vi "n set piso control.vi"(8 "error in (no error)":errorcluster, 9 "l2":u16, 10 "l1":u16, 11 "n":u16) -> (0 "error out":errorcluster)   [LabVIEW 2015, in "SCANalone4x64.lvlib"]
doc: "__declspec(dllimport) void __stdcall n_set_piso_control(unsigned short n, unsigned short l1, unsigned short l2);"
uses:
  <userlib>/SCANalone4x64/SCANalone4x64.lvlib
  <userlib>/SCANalone4x64/SCANalone4x64.dll
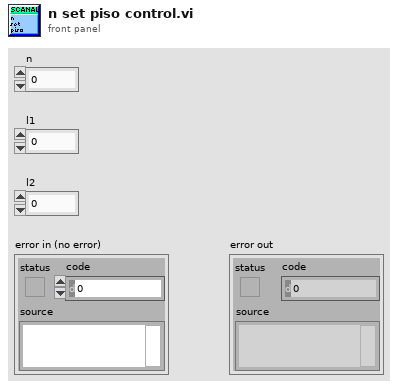
[diagram p1: front panel]
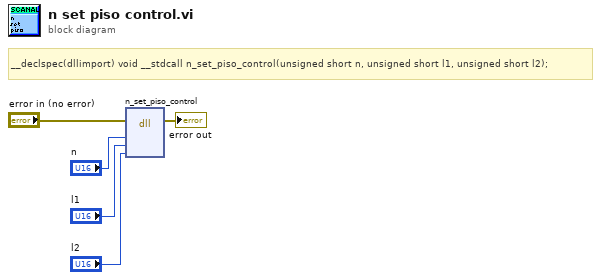
[diagram p0: block diagram]
diagram:
  # "__declspec(dllimport) void __stdcall n_set_piso_control(unsigned short n, unsigned short l1, unsigned short l2);"
  n1 = dll-call lib="C:/Program Files/National Instruments/LabVIEW 2015/user.lib/SCANalone4x64/SCANalone4x64.*" fn="n_set_piso_control"(error in="error in (no error)", "n"="n", "l1"="l1", "l2"="l2") -> (error out=→"error out":errorcluster)  [unwired: 6 in, 1 out]
